vi "DLPVA_4_ReadAll.vi"() -> (6 "gain 1":bool, 8 "gain 2":bool, 10 "coupling":bool, 15 "filter":bool)   [LabVIEW 2013]
panel:
  # "4"
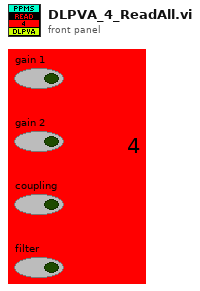
[diagram p1: front panel]
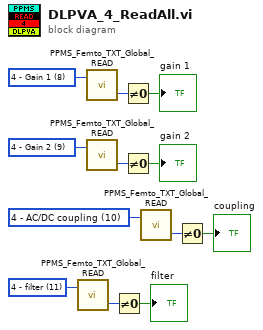
[diagram p0: block diagram]
diagram:
  w10 = u16 11 items=["1 - DDPCA Gain (V/A)", "2 - DDPCA Gain (V/A)", "3 - DLPVA Gain (dB)", "3 - Gain 1", "3 - Gain 2", "3 - AC/DC coupling", "3 - filter", "4 - DLPVA Gain (dB)", "4 - Gain 1", "4 - Gain 2", "4 - AC/DC coupling", "4 - filter"] ("Property")
  w11 = u16 10 items=["1 - DDPCA Gain (V/A)", "2 - DDPCA Gain (V/A)", "3 - DLPVA Gain (dB)", "3 - Gain 1", "3 - Gain 2", "3 - AC/DC coupling", "3 - filter", "4 - DLPVA Gain (dB)", "4 - Gain 1", "4 - Gain 2", "4 - AC/DC coupling", "4 - filter"] ("Property")
  w12 = u16 9 items=["1 - DDPCA Gain (V/A)", "2 - DDPCA Gain (V/A)", "3 - DLPVA Gain (dB)", "3 - Gain 1", "3 - Gain 2", "3 - AC/DC coupling", "3 - filter", "4 - DLPVA Gain (dB)", "4 - Gain 1", "4 - Gain 2", "4 - AC/DC coupling", "4 - filter"] ("Property")
  w9 = u16 8 items=["1 - DDPCA Gain (V/A)", "2 - DDPCA Gain (V/A)", "3 - DLPVA Gain (dB)", "3 - Gain 1", "3 - Gain 2", "3 - AC/DC coupling", "3 - filter", "4 - DLPVA Gain (dB)", "4 - Gain 1", "4 - Gain 2", "4 - AC/DC coupling", "4 - filter"] ("Property")
  n1 = call "PPMS_Femto_TXT_Global_READ.vi"("Property"=w10) -> ("Value"=w5:i32)  [unwired: 1 in, 1 out]
  n2 = call "PPMS_Femto_TXT_Global_READ.vi"("Property"=w9) -> ("Value"=w2:i32)  [unwired: 1 in, 1 out]
  n3 = call "PPMS_Femto_TXT_Global_READ.vi"("Property"=w12) -> ("Value"=w1:i32)  [unwired: 1 in, 1 out]
  n4 = Not Equal To 0?(x=w5) -> (x != 0?=→"filter":bool)
  n5 = Not Equal To 0?(x=w2) -> (x != 0?=→"gain 1":bool)
  n6 = Not Equal To 0?(x=w1) -> (x != 0?=→"gain 2":bool)
  n7 = call "PPMS_Femto_TXT_Global_READ.vi"("Property"=w11) -> ("Value"=w4:i32)  [unwired: 1 in, 1 out]
  n8 = Not Equal To 0?(x=w4) -> (x != 0?=→"coupling":bool)
